vi "Read Overlay colors.vi"(8 "error in (no error)":errorcluster, 11 "Overlay Base in":refnum<class "Analyze Results Base.lvclass">) -> (0 "error out":errorcluster, 2 "Overlay colors":cluster{"Border":u32, "Text":u32}={"Border"=16448250, "Text"=16448250}, 3 "Overlay Base out":refnum<class "Analyze Results Base.lvclass">)   [LabVIEW 2014, in "Analyze Results Base.lvclass"]
uses:
  Analyze Results Base.lvclass
  Analyze Results Base.lvclass/Analyze Results Base.ctl
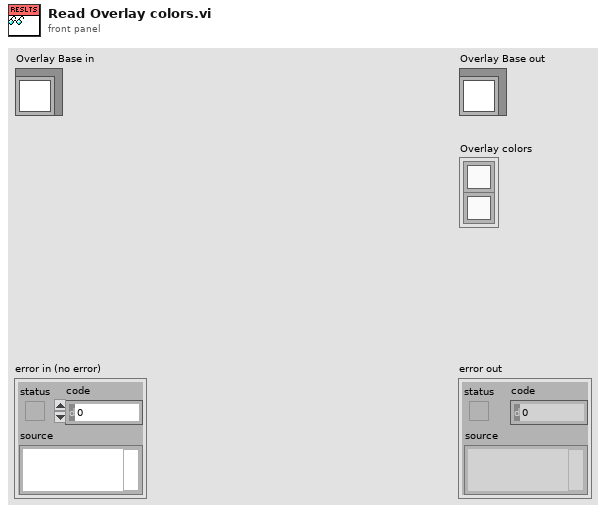
[diagram p1: front panel]
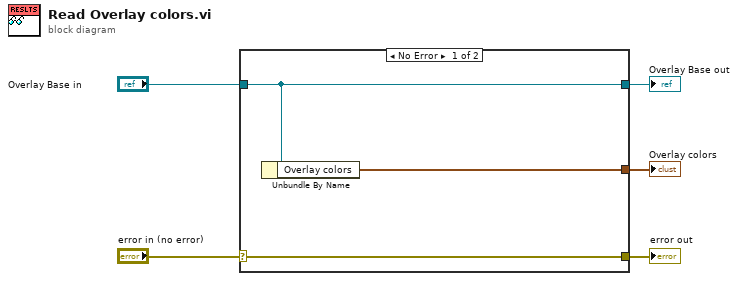
[diagram p0: block diagram]
diagram:
  n1 = case shown="No Error" "error in (no error)" {
    selector: "error in (no error)" -> [w8 w9]
    tunnel: [w8 w9] -> w4
    tunnel: [w7 w10] -> w2
    tunnel: "Overlay Base in" -> [w7 w10]
    tunnel: [w6 _] -> w1
    frame No Error {
      n2 = Unbundle By Name(w7) -> ("Overlay colors"=w6:cluster{"Border":u32, "Text":u32})
    }
    frame Error {
    }
  }
  "error out" <- w4
  "Overlay Base out" <- w2
  "Overlay colors" <- w1
